vi "HungarianMethod.vi"(11 "Processing Time Matrix":i32[][](array[numeric])=[[85, 23, 39, 55], [85, 74, 56, 78], [3, 96, 92, 11], [67, 45, 70, 75]]) -> (2 "cost":dbl, 3 "Assignment":i8[][](array[numeric]))   [LabVIEW 2013]
uses:
  <vilib>/Analysis/Matrix/Datatypes/RealMatrix.ctl
  <vilib>/Analysis/Matrix/Numeric/Conversions/Array To Matrix - RA2.vi
  <vilib>/Analysis/Matrix/Numeric/Conversions/Matrix To Array - RM.vi
  <vilib>/Analysis/Matrix/NI_Matrix.lvlib
panel:
  out "Munkres Matrix":T1
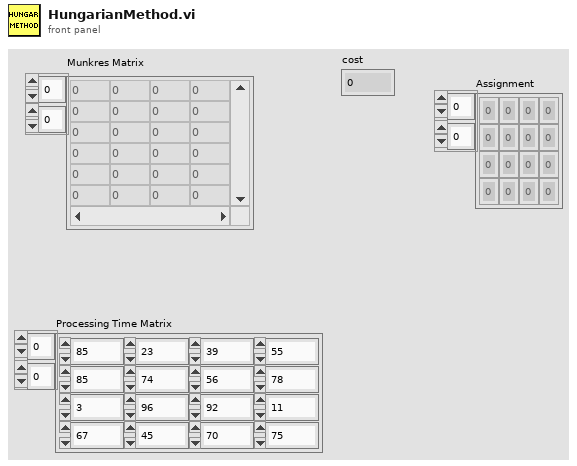
[diagram p1: front panel]
types:
  T1 = typedef "NI_Matrix.lvlib/RealMatrix.ctl" = dbl[][]
  T2 = enum16{"Step 1", "Step 2", "Step 3", "Step 4", "Step 5", "Step 6"}
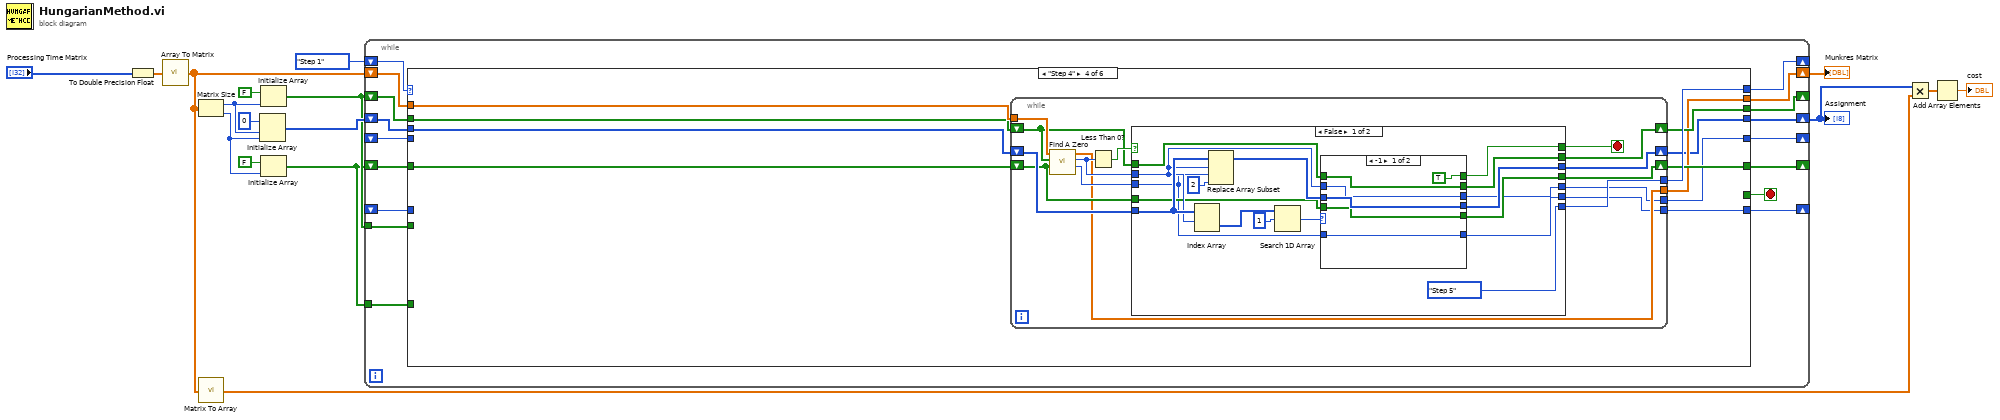
[diagram p0: block diagram]
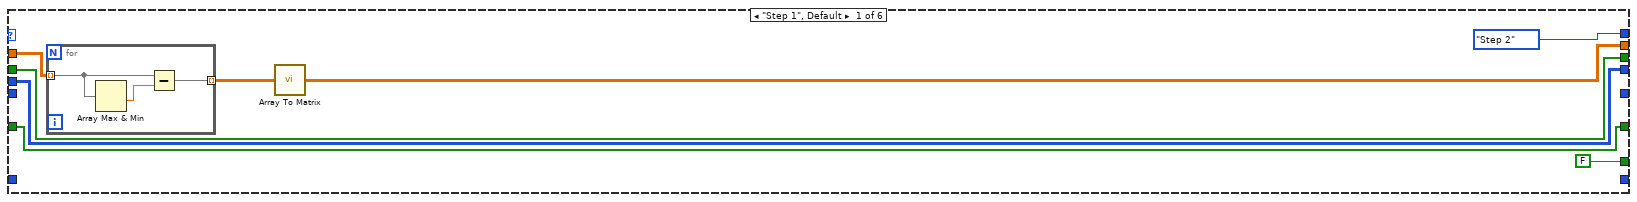
[diagram p2: hidden frame]
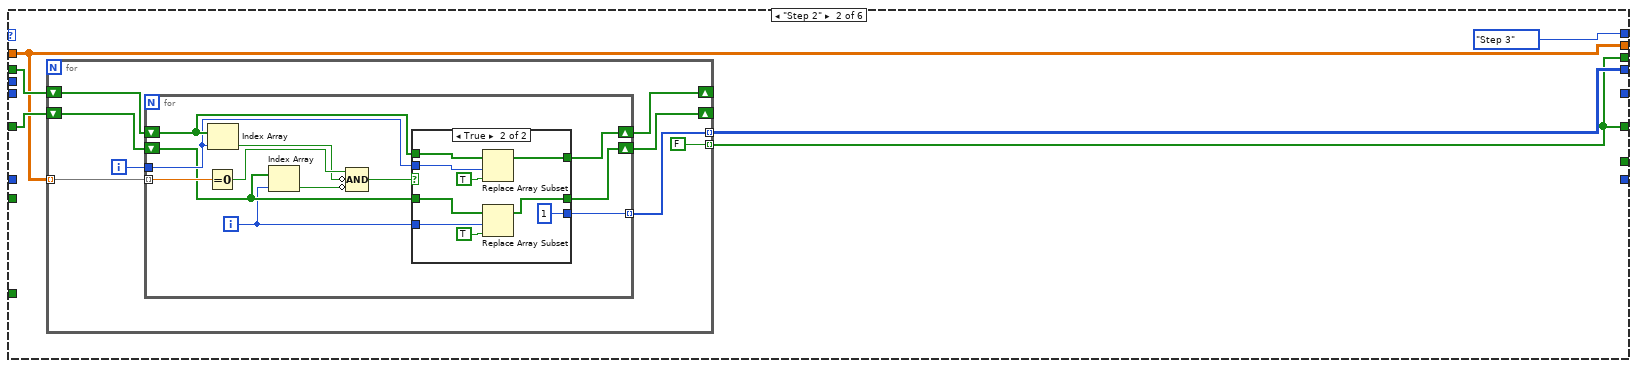
[diagram p3: hidden frame]
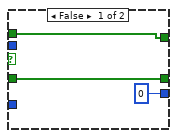
[diagram p4: hidden frame]
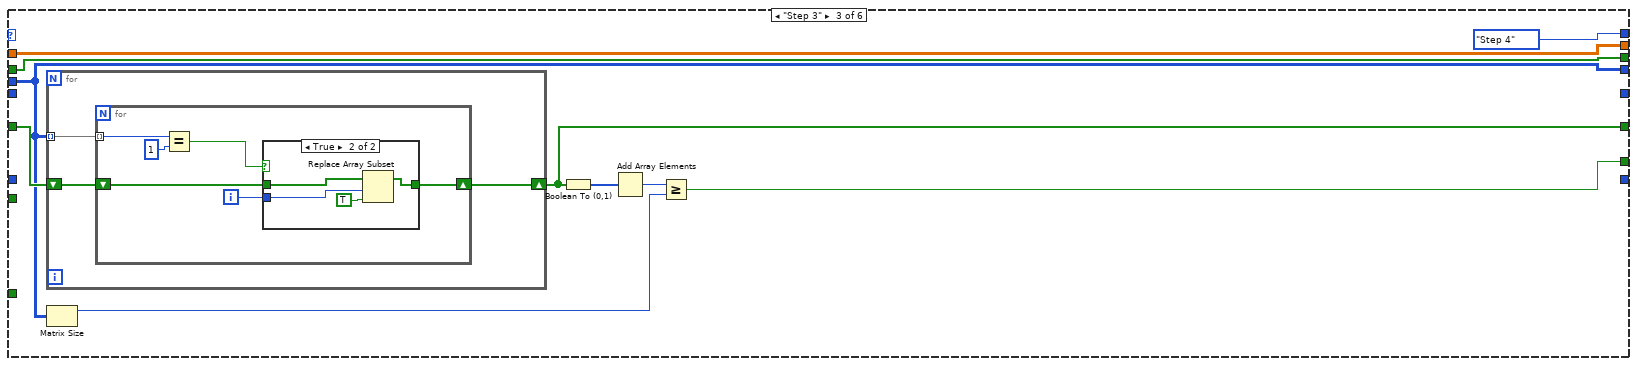
[diagram p5: hidden frame]
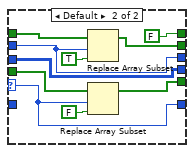
[diagram p7: hidden frame]
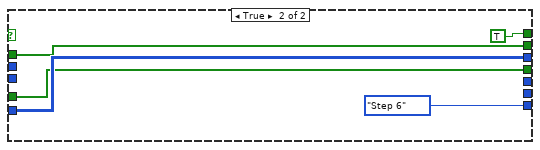
[diagram p8: hidden frame]
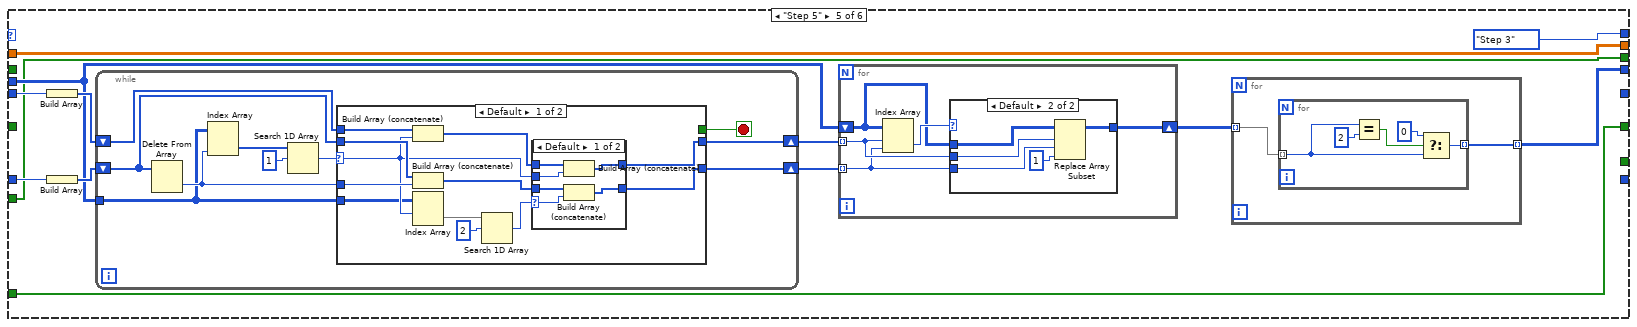
[diagram p9: hidden frame]
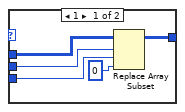
[diagram p10: hidden frame]
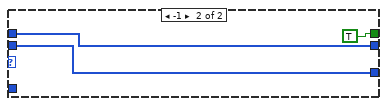
[diagram p12: hidden frame]
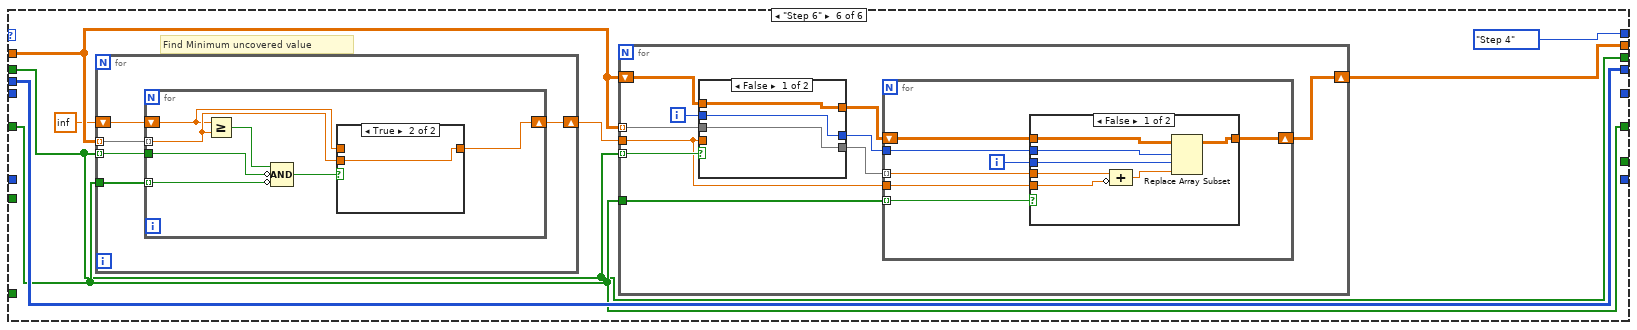
[diagram p13: hidden frame]
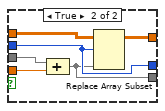
[diagram p14: hidden frame]
diagram:
  n1 = To Double Precision Float(number="Processing Time Matrix") -> (double precision float=w1:dbl[][])
  n2 = call-poly <vilib>:"Array To Matrix.vi"("Real 2D Array"=w1) -> ("Real Matrix"=w3:T1)
  n3 = Matrix Size(0:w3) -> (1:w13:i32, 2:w14:i32)
  n4 = call-poly <vilib>:"Matrix To Array.vi"("Real Matrix"=w3) -> ("Real 2D Array"=w7:dbl[][])
  n5 = Initialize Array(i8 0, w13, w14) -> (w11:i8[][])
  n6 = Initialize Array(FALSE, w13) -> (w10:bool[])
  n7 = Initialize Array(FALSE, w14) -> (w9:bool[])
  n8 = while {
    shift-right: [w18] -> _
    shift-left: T2."Step 1" -> [w34]
    shift-right: [w31] -> w8
    shift-left: w3 -> [w32]
    shift-right: [w26] -> _
    shift-left: w10 -> [w30]
    shift-right: [w27] -> _
    shift-left: w9 -> [w29]
    shift-right: [w28] -> w6
    shift-left: w11 -> [w25]
    shift-right: [w23] -> _
    shift-left: _ -> [w22]
    shift-right: [w24] -> _
    shift-left: _ -> [w21]
    tunnel: w10 -> [w20]
    tunnel: w9 -> [w19]
    stop <- w33 stop-if-true
    n9 = case shown="\"Step 4\"" w34 {
      tunnel: [FALSE _ w85 _ _ _] -> w33
      tunnel: w32 -> [w41 w47 w93 w118 w179 w245]
      tunnel: [w39 w47 w93 w111 w179 w243] -> w31
      tunnel: [T2."Step 2" T2."Step 3" T2."Step 4" w114 T2."Step 3" T2."Step 4"] -> w18
      tunnel: w30 -> [w37 w50 w89 w117 _ w241]
      tunnel: w29 -> [w36 w49 w92 w116 _ w242]
      tunnel: [w35 w48 w88 w110 w172 w246] -> w28
      tunnel: [w36 w46 w90 w113 w174 w242] -> w27
      tunnel: [w37 w46 w89 w112 w175 w241] -> w26
      tunnel: w25 -> [w35 _ w88 w115 w178 w246]
      tunnel: [_ _ _ w109 _ _] -> w24
      tunnel: [_ _ _ w108 _ _] -> w23
      tunnel: w22 -> [_ _ _ _ w183 _]
      tunnel: w21 -> [_ _ _ _ w182 _]
      tunnel: w20 -> [_ _ _ _ w175 _]
      tunnel: w19 -> [_ _ _ _ w174 _]
      frame "Step 1", Default {
        n10 = for {
          tunnel: w41 -> [w44] mode=indexing
          tunnel: [w43] -> w40 mode=indexing
          n11 = Array Max & Min(array=w44) -> (min value=w45:dbl)  [unwired: 3 out]
          n12 = Subtract(x=w44, y=w45) -> (x-y=w43:dbl[])
        }
        n13 = call-poly <vilib>:"Array To Matrix.vi"("Real 2D Array"=w40) -> ("Real Matrix"=w39:T1)
      }
      frame "Step 2" {
        n14 = for {
          tunnel: w47 -> [w59] mode=indexing
          shift-right: [w55] -> _
          shift-left: w50 -> [w58]
          shift-right: [w54] -> _
          shift-left: w49 -> [w57]
          tunnel: [w53] -> w48 mode=indexing
          tunnel: [FALSE] -> w46 mode=indexing
          i -> [w56]
          n15 = for {
            tunnel: w59 -> [w71] mode=indexing
            shift-right: [w64] -> w55
            shift-left: w58 -> [w66]
            shift-right: [w61] -> w54
            shift-left: w57 -> [w63]
            tunnel: w56 -> [w65]
            tunnel: [w60] -> w53 mode=indexing
            i -> [w62]
            n16 = Equal To 0?(x=w71) -> (x = 0?=w70:bool)
            n17 = Index Array(array=w66, index=w65) -> (element=w69:bool)
            n18 = Index Array(array=w63, index=w62) -> (element=w68:bool)
            n19 = Compound Arithmetic op=AND(w70, invert w69, invert w68) -> (w67:bool)
            n20 = case shown="True" w67 {
              tunnel: w66 -> [w74 w83]
              tunnel: w65 -> [_ w82]
              tunnel: [w74 w81] -> w64
              tunnel: w63 -> [w73 w80]
              tunnel: w62 -> [_ w79]
              tunnel: [w73 w76] -> w61
              tunnel: [i8 0 i8 1] -> w60
              frame False {
              }
              frame True {
                n21 = Replace Array Subset(array=w83, new element=TRUE ("new element/subarray"), index=w82) -> (w81:bool[])
                n22 = Replace Array Subset(array=w80, new element=TRUE ("new element/subarray"), index=w79) -> (w76:bool[])
              }
            }
          }
        }
      }
      frame "Step 3" {
        n23 = for {
          tunnel: w88 -> [w96] mode=indexing
          shift-right: [w94] -> w90
          shift-left: w92 -> [w95]
          n24 = for {
            tunnel: w96 -> [w102] mode=indexing
            shift-right: [w97] -> w94
            shift-left: w95 -> [w99]
            i -> [w98]
            n25 = Equal?(x=w102, y=i8 1) -> (x = y?=w100:bool)
            n26 = case shown="True" w100 {
              tunnel: w99 -> [w103 w107]
              tunnel: w98 -> [_ w106]
              tunnel: [w103 w104] -> w97
              frame False {
              }
              frame True {
                n27 = Replace Array Subset(array=w107, new element=TRUE ("new element/subarray"), index=w106) -> (w104:bool[])
              }
            }
          }
        }
        n28 = Matrix Size(0:w88) -> (1:w86:i32)  [unwired: 1 out]
        n29 = Boolean To (0,1)(Boolean=w90) -> (0, 1=w91:i16[])
        n30 = Add Array Elements(numeric array=w91) -> (sum=w87:i16)
        n31 = Greater Or Equal?(x=w87, y=w86) -> (x >= y?=w85:bool)
      }
      frame "Step 4" {
        n32 = while {
          tunnel: w118 -> [w133]
          shift-right: [w127] -> w112
          shift-left: w117 -> [w126]
          shift-right: [w129] -> w113
          shift-left: w116 -> [w128]
          shift-right: [w130] -> w110
          shift-left: w115 -> [w131]
          tunnel: [w125] -> w114
          tunnel: [w121] -> w111
          tunnel: [w119] -> w109
          tunnel: [w120] -> w108
          stop <- w122 stop-if-true
          n33 = call "Find A Zero.vi"("Ccovered"=w128, "Rcovered"=w126, "Matrix"=w133) -> ("Column"=w124:i32, "Row"=w123:i32, "Matrix Out"=w121:T1)  [unwired: 6 in]
          n34 = Less Than 0?(x=w123) -> (x < 0?=w132:bool)
          n35 = case shown="False" w132 {
            tunnel: w131 -> [w149 w171]
            tunnel: [w144 w171] -> w130
            tunnel: [w138 w170] -> w129
            tunnel: w128 -> [w137 w170]
            tunnel: [w139 w169] -> w127
            tunnel: w126 -> [w141 w169]
            tunnel: [T2."Step 5" T2."Step 6"] -> w125
            tunnel: w124 -> [w134 _]
            tunnel: w123 -> [w140 _]
            tunnel: [w145 TRUE] -> w122
            tunnel: [w136 _] -> w119
            tunnel: [w135 _] -> w120
            frame False {
              n36 = Index Array(array=w149, index (row)=w140) -> (element=w148:i8[])  [unwired: 1 in]
              n37 = Replace Array Subset(array=w149, new element=i8 2 ("new element/subarray"), index (row)=w140, index (col)=w134) -> (w143:i8[][])
              n38 = Search 1D Array(1D array=w148, element=i8 1) -> (index of element=w146:i32)  [unwired: 1 out]
              n39 = case shown="-1" w146 {
                selector: w146 -> [_ w158]
                tunnel: [TRUE FALSE] -> w145
                tunnel: [w155 w165] -> w144
                tunnel: w143 -> [w155 w165]
                tunnel: w141 -> [w154 w164]
                tunnel: w140 -> [w152 w157]
                tunnel: [w154 w162] -> w139
                tunnel: [w153 w160] -> w138
                tunnel: w137 -> [w153 w159]
                tunnel: [w151 w158] -> w136
                tunnel: [w152 w157] -> w135
                tunnel: w134 -> [w151 _]
                frame -1 {
                }
                frame Default {
                  n40 = Replace Array Subset(array=w164, new element=TRUE ("new element/subarray"), index=w157) -> (w162:bool[])
                  n41 = Replace Array Subset(array=w159, new element=FALSE ("new element/subarray"), index=w158) -> (w160:bool[])
                }
              }
            }
            frame True {
            }
          }
        }
      }
      frame "Step 5" {
        n42 = Build Array(w183) -> (w184:i32[])
        n43 = Build Array(w182) -> (w181:i32[])
        n44 = while {
          shift-right: [w212] -> w177
          shift-left: w184 -> [w211]
          shift-right: [w210] -> w176
          shift-left: w181 -> [w209]
          tunnel: w178 -> [w207]
          stop <- w213 stop-if-true
          n45 = Delete From Array(array=w209) -> (deleted portion=w208:i32)  [unwired: 2 in, 1 out]
          n46 = Index Array(array=w207, index (col)=w208) -> (element=w216:i8[])  [unwired: 1 in]
          n47 = Search 1D Array(1D array=w216, element=i8 1) -> (index of element=w214:i32)  [unwired: 1 out]
          n48 = case shown="Default" w214 {
            selector: w214 -> [w218 _]
            tunnel: [_ TRUE] -> w213
            tunnel: [w222 w238] -> w212
            tunnel: w211 -> [w228 w238]
            tunnel: [w220 w237] -> w210
            tunnel: w209 -> [w227 w237]
            tunnel: w208 -> [w226 _]
            tunnel: w207 -> [w217 _]
            frame Default {
              n49 = Build Array (concatenate)(w228, w218) -> (w221:i32[])
              n50 = Build Array (concatenate)(w227, w226) -> (w219:i32[])
              n51 = Index Array(array=w217, index (row)=w218) -> (element=w224:i8[])  [unwired: 1 in]
              n52 = Search 1D Array(1D array=w224, element=i8 2) -> (index of element=w223:i32)  [unwired: 1 out]
              n53 = case shown="Default" w223 {
                selector: w223 -> [w229 _]
                tunnel: [w232 w236] -> w222
                tunnel: w221 -> [w234 w236]
                tunnel: [w231 w235] -> w220
                tunnel: w219 -> [w230 w235]
                tunnel: w218 -> [w233 _]
                frame Default {
                  n54 = Build Array (concatenate)(w234, w233) -> (w232:i32[])
                  n55 = Build Array (concatenate)(w230, w229) -> (w231:i32[])
                }
                frame -1 {
                }
              }
            }
            frame -1 {
            }
          }
        }
        n56 = for {
          shift-right: [w194] -> w173
          shift-left: w178 -> [w195]
          tunnel: w177 -> [w193] mode=indexing
          tunnel: w176 -> [w192] mode=indexing
          n57 = Index Array(array=w195, index (row)=w193, index (col)=w192) -> (element=w196:i8)
          n58 = case shown="Default" w196 {
            tunnel: w195 -> [w201 w206]
            tunnel: [w200 w205] -> w194
            tunnel: w193 -> [w199 w204]
            tunnel: w192 -> [w198 w203]
            frame 1 {
              n59 = Replace Array Subset(array=w201, new element=i8 0 ("new element/subarray"), index (row)=w199, index (col)=w198) -> (w200:i8[][])
            }
            frame Default {
              n60 = Replace Array Subset(array=w206, new element=i8 1 ("new element/subarray"), index (row)=w204, index (col)=w203) -> (w205:i8[][])
            }
          }
        }
        n61 = for {
          tunnel: w173 -> [w186] mode=indexing
          tunnel: [w185] -> w172 mode=indexing
          n62 = for {
            tunnel: w186 -> [w187] mode=indexing
            tunnel: [w189] -> w185 mode=indexing
            n63 = Equal?(x=w187, y=i8 2) -> (x = y?=w190:bool)
            n64 = Select(t=i8 0 ("f"), s=w190, f=w187) -> (s? t:f=w189:i8)
          }
        }
      }
      frame "Step 6" {
        # "Find Minimum uncovered value"
        n65 = for {
          tunnel: w245 -> [w286] mode=indexing
          shift-right: [w282] -> w244
          shift-left: inf ("Real Matrix Element") -> [w285]
          tunnel: w241 -> [w284] mode=indexing
          tunnel: w242 -> [w283]
          n66 = for {
            tunnel: w286 -> [w289] mode=indexing
            tunnel: w284 -> [w292]
            tunnel: w283 -> [w291] mode=indexing
            shift-right: [w288] -> w282
            shift-left: w285 -> [w287]
            n67 = Greater Or Equal?(x=w287, y=w289) -> (x >= y?=w293:bool)
            n68 = Compound Arithmetic op=AND(w293, invert w292, invert w291) -> (w290:bool)
            n69 = case shown="True" w290 {
              tunnel: w289 -> [_ w295]
              tunnel: [w294 w295] -> w288
              tunnel: w287 -> [w294 _]
              frame False {
              }
              frame True {
              }
            }
          }
        }
        n70 = for {
          tunnel: w242 -> [w254]
          tunnel: w241 -> [w255] mode=indexing
          shift-right: [w250] -> w243
          shift-left: w245 -> [w257]
          tunnel: w245 -> [w249] mode=indexing
          tunnel: w244 -> [w252]
          i -> [w256]
          n71 = case shown="False" w255 {
            tunnel: w257 -> [w260 w266]
            tunnel: w256 -> [w259 w262]
            tunnel: w249 -> [w258 w265]
            tunnel: w252 -> [_ w264]
            tunnel: [w260 w263] -> w251
            tunnel: [w259 w262] -> w253
            tunnel: [w258 w261] -> w248
            frame False {
            }
            frame True {
              n72 = Compound Arithmetic op=ADD(w265, w264) -> (w261:dbl[])
              n73 = Replace Array Subset(array=w266, new element=w261, index (row)=w262) -> (w263:T1)  [unwired: 1 in]
            }
          }
          n74 = for {
            tunnel: w254 -> [w273] mode=indexing
            shift-right: [w267] -> w250
            shift-left: w251 -> [w272]
            tunnel: w248 -> [w271] mode=indexing
            tunnel: w252 -> [w270]
            tunnel: w253 -> [w268]
            i -> [w269]
            n75 = case shown="False" w273 {
              tunnel: w272 -> [w280 w281]
              tunnel: w271 -> [w278 _]
              tunnel: w270 -> [w279 _]
              tunnel: w269 -> [w276 _]
              tunnel: w268 -> [w274 _]
              tunnel: [w275 w281] -> w267
              frame False {
                n76 = Compound Arithmetic op=ADD(w278, invert w279) -> (w277:dbl)
                n77 = Replace Array Subset(array=w280, new element=w277, index (row)=w274, index (col)=w276) -> (w275:T1)
              }
              frame True {
              }
            }
          }
        }
      }
    }
  }
  "Munkres Matrix" <- w8
  "Assignment" <- w6
  n78 = Multiply(x=w6, y=w7) -> (x*y=w5:dbl[][])
  n79 = Add Array Elements(numeric array=w5) -> (sum=→"cost":dbl)
